vi "Counter.vi"(2 "error in":errorcluster caption="error in (no error)", 3 "Time Target (s)":dbl=1800.0 format="%#_13g") -> (0 "error out":errorcluster, 1 "倒數時間":string)   [LabVIEW 2019]
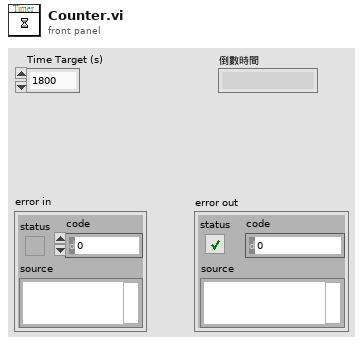
[diagram p1: front panel]
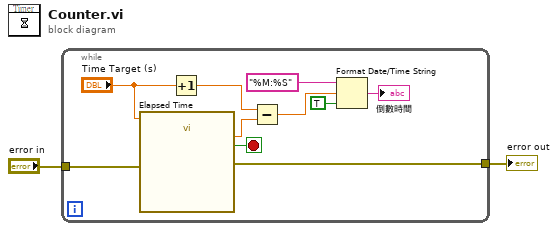
[diagram p0: block diagram]
diagram:
  n1 = while {
    tunnel: "error in" -> [w12]
    tunnel: [w3] -> w1
    stop <- w4 stop-if-true
    n2 = call "Elapsed Time"("Time Target (s)"="Time Target (s)", "error in (no error)"=w12) -> ("Elapsed Time (s)"=w9:dbl, "Time has Elapsed"=w4:bool, "error out"=w3:errorcluster)  [unwired: 10 in, 5 out]
    n3 = Increment(x="Time Target (s)") -> (x+1=w10:dbl)
    n4 = Subtract(x=w10, y=w9) -> (x-y=w7:dbl)
    n5 = Format Date/Time String(time format string (%c)="%M:%S", seconds (now)=w7, UTC format=TRUE) -> (date/time string=→"倒數時間":string)
  }
  "error out" <- w1
